vi "Log_PACKET - Add Packet to Queue.vi"(1 "Complete Packet":T1 {"Packet Data" format="%.0x"}, 12 "error in (no error)":errorcluster, 13 "TX? (F: RX)":bool) -> (3 "Complete Packet dup":T1 {"Packet Data" format="%.0x"}, 14 "error out":errorcluster)   [LabVIEW 2014]
uses:
  PacketMode/SRV_PM_Packet.ctl
panel:
  out "TX Packet String dup":string
  in  "TX Packet String":string
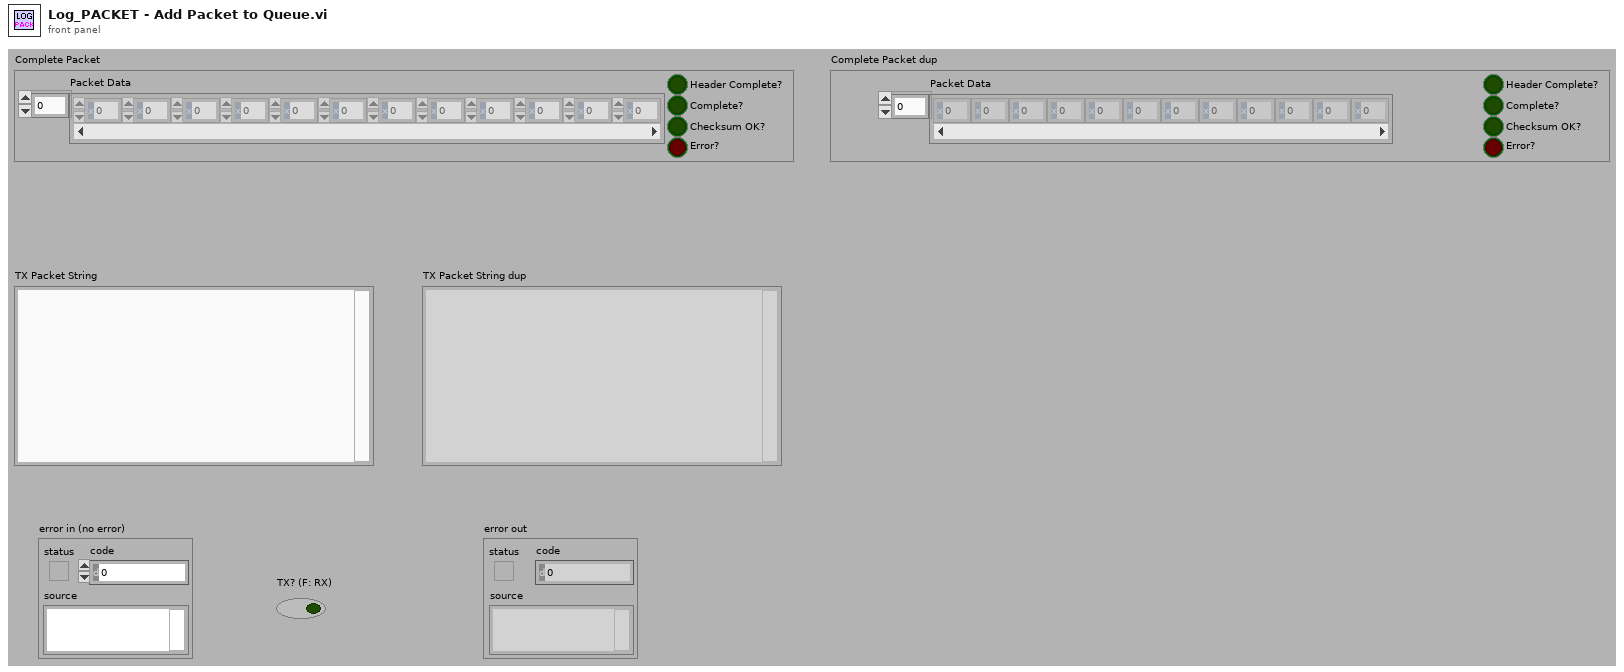
[diagram p1: front panel]
types:
  T1 = typedef "SRV_PM_Packet.ctl" = cluster{"Packet Data":u8[], "Header Complete?":bool, "Complete?":bool, "Checksum OK?":bool, "Error?":bool}
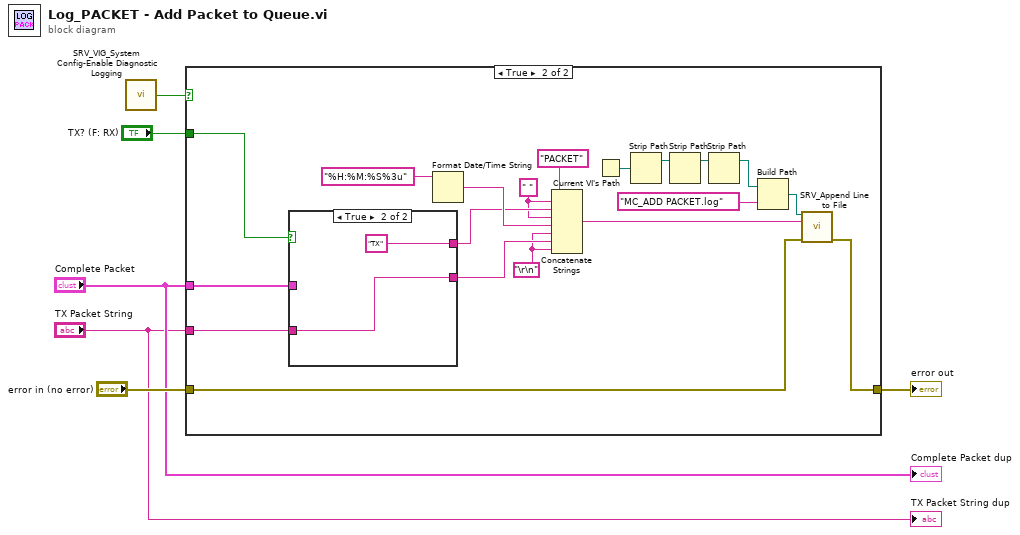
[diagram p0: block diagram]
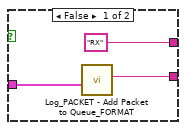
[diagram p3: hidden frame]
diagram:
  n1 = call "SRV_VIG_System Config-Enable Diagnostic Logging.vi"() -> ("Enable Diagnostic Log?"=w1:bool)  [unwired: 15 in]
  n2 = case shown="True" w1 {
    tunnel: [w7 w24] -> w6
    tunnel: "error in (no error)" -> [w7 w23]
    tunnel: "Complete Packet" -> [_ w14]
    tunnel: "TX? (F: RX)" -> [_ w12]
    tunnel: "TX Packet String" -> [_ w11]
    frame False {
    }
    frame True {
      w13 = "\r\n"
      w8 = " " ("string")
      n3 = case shown="True" w12 {
        tunnel: [w29 w31] -> w15
        tunnel: w14 -> [w28 _]
        tunnel: w11 -> [_ w31]
        tunnel: ["RX" "TX"] -> w10
        frame False {
          n4 = call "Log_PACKET - Add Packet to Queue_FORMAT.vi"("Complete Packet"=w28) -> ("resulting string"=w29:string)  [unwired: 10 in]
        }
        frame True {
        }
      }
      n5 = Format Date/Time String(time format string (%c)="%H:%M:%S%3u") -> (date/time string=w16:string)  [unwired: 2 in]
      n6 = Concatenate Strings("PACKET" ("string"), w8, w10, w8, w16, w13, w15, w13) -> (w25:string)
      n7 = Current VI's Path() -> (path=w18:path)
      n8 = Strip Path(path=w18) -> (stripped path=w19:path)  [unwired: 1 out]
      n9 = Strip Path(path=w19) -> (stripped path=w20:path)  [unwired: 1 out]
      n10 = Strip Path(path=w20) -> (stripped path=w17:path)  [unwired: 1 out]
      n11 = Build Path(base path=w17, name or relative path="MC_ADD PACKET.log") -> (appended path=w21:path)
      n12 = call "SRV_Append Line to File.vi"("file path"=w21, "Line to Write"=w25, "error in (no error)"=w23) -> ("error out"=w24:errorcluster)  [unwired: 12 in]
    }
  }
  "error out" <- w6
  "Complete Packet dup" <- "Complete Packet"
  "TX Packet String dup" <- "TX Packet String"
